vi "Inline or Forked.vi"(8 "error in (no error)":errorcluster, 9 "Inline or Forked":T1, 10 "Assert VI Path":path, 11 "Wire in":refnum<vi>) -> (0 "error out":errorcluster, 2 "New Node Ref":refnum<vi>)   [LabVIEW 2017]
uses:
  Inline or Forked.ctl
  <vilib>/_script/New VI Object TypeDefs/NewVIObject_LVRelativePositionTypeDef.ctl
  <vilib>/_script/New VI Object TypeDefs/NewVIObject_LVRelativeDirectionTypeDef.ctl
  <vilib>/Utility/miscctls.llb/LVPoint32TypeDef.ctl
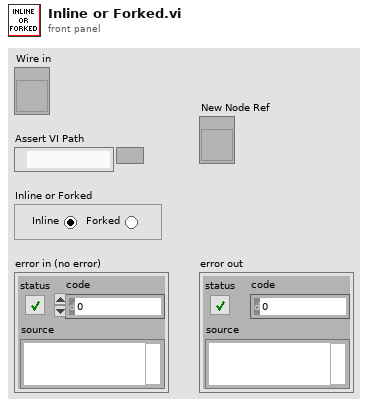
[diagram p1: front panel]
types:
  T1 = typedef "Inline or Forked.ctl" = enum32{"Inline", "Forked"}
  T2 = typedef "NewVIObject_LVRelativeDirectionTypeDef.ctl" = enum32{"Right", "Left", "Top", "Bottom", "Top Right", "Top Left", "Bottom Right", "Bottom Left"}
  T3 = typedef "LVPoint32TypeDef.ctl" = cluster{"Horizontal":i32, "Vertical":i32}
  T4 = typedef "NewVIObject_LVRelativePositionTypeDef.ctl" = cluster{"Refnum":refnum<vi>, "Relative Direction":T2, "Point32":T3}
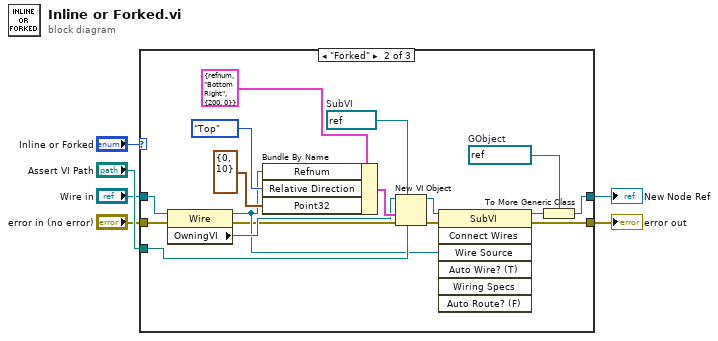
[diagram p0: block diagram]
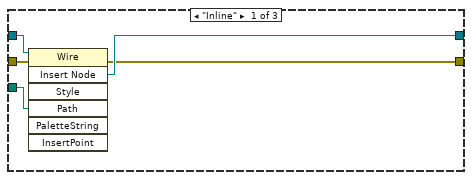
[diagram p2: hidden frame]
diagram:
  n1 = case shown="\"Forked\"" "Inline or Forked" {
    tunnel: [w11 w13 _] -> w6
    tunnel: "Assert VI Path" -> [w10 w21 _]
    tunnel: "Wire in" -> [w9 w28 _]
    tunnel: [w8 w15 _] -> w3
    tunnel: "error in (no error)" -> [w7 w16 _]
    frame "Inline" {
      n2 = invoke class="Wire" method="Insert Node"(reference=w9, error in=w7, "Path"=w10) -> (error out=w8:errorcluster, "Insert Node"=w11:refnum<vi>)  [unwired: 4 in, 5 out]
    }
    frame "Forked" {
      w12 = refnum<vi> refnum  # GObject
      w27 = refnum<vi> refnum  # SubVI
      n3 = property class="Wire"(reference=w28, error in=w16) -> (reference out=w19:refnum<vi>, error out=w17:errorcluster, "OwningVI"=w22:refnum<vi>)
      n4 = Bundle By Name(cluster=T4 {"Refnum"=refnum, "Relative Direction"=enum."Bottom Right", "Point32"={"Horizontal"=200, "Vertical"=0}} ("Relative Position"), "Refnum"=w19, "Relative Direction"=NewVIObject_LVRelativeDirectionTypeDef."Top", "Point32"=T3 {"Horizontal"=0, "Vertical"=10}) -> (w23:T4)
      n5 = New VI Object(vi object class=w27, owner refnum=w22, position/next to=w23, 6:w21, 8:w17) -> (object refnum=w20:refnum<vi>, 0:w18:errorcluster)  [unwired: 3 in]
      n6 = invoke class="SubVI" method="Connect Wires"(reference=w20, error in=w18, "Wire Source"=w19) -> (reference out=w14:refnum<vi>, error out=w15:errorcluster)  [unwired: 4 in, 5 out]
      n7 = To More Generic Class(target class=w12, reference=w14) -> (generic class reference=w13:refnum<vi>)
    }
    frame Default {
    }
  }
  "New Node Ref" <- w6
  "error out" <- w3
